vi "Z.vi"(8 "error in (no error)":errorcluster, 10 "Wire in":T1, 11 "Gate in":refnum<class "G-UE.lvclass">) -> (0 "error out":errorcluster, 3 "Gate out":refnum<class "G-UE.lvclass">)   [LabVIEW 2016, in "G-UE.lvclass"]
uses:
  G-UE.lvclass
  TypeDefs/Circuit Cluster.ctl
  GateAbst/GateAbst.lvclass
  <vilib>/Analysis/Matrix/Datatypes/ComplexMatrix.ctl
  <vilib>/Analysis/Matrix/NI_Matrix.lvlib
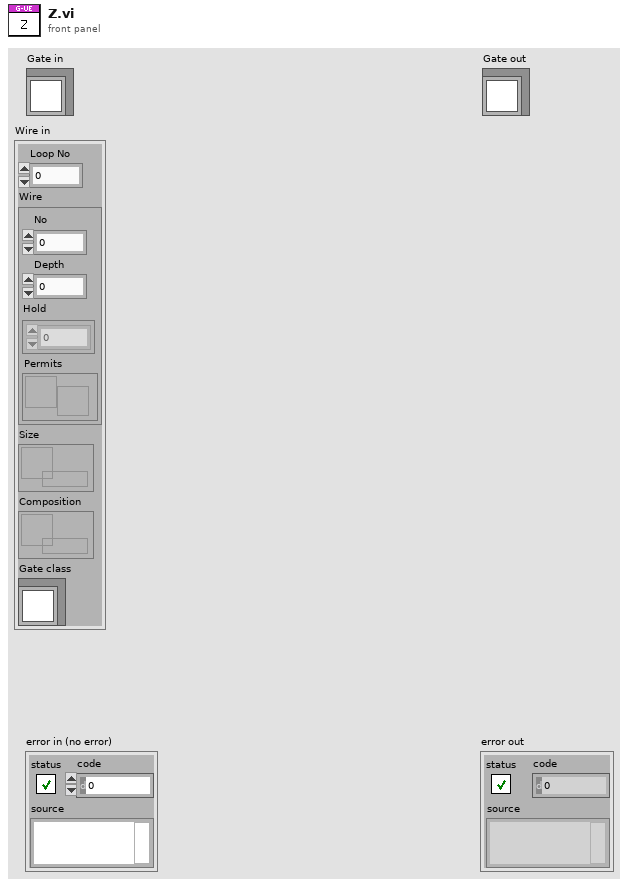
[diagram p1: front panel]
types:
  T1 = typedef "Circuit Cluster.ctl" = cluster{"Loop No":i32, "Wire":cluster{"No":i32, "Depth":i32, "Hold":i32[][], "Permits":refnum<notifier>}, "Size":refnum<queue>, "Composition":refnum<queue>, "Gate class":refnum<class "GateAbst.lvclass">}
  T2 = typedef "NI_Matrix.lvlib/ComplexMatrix.ctl" = cdb[][]
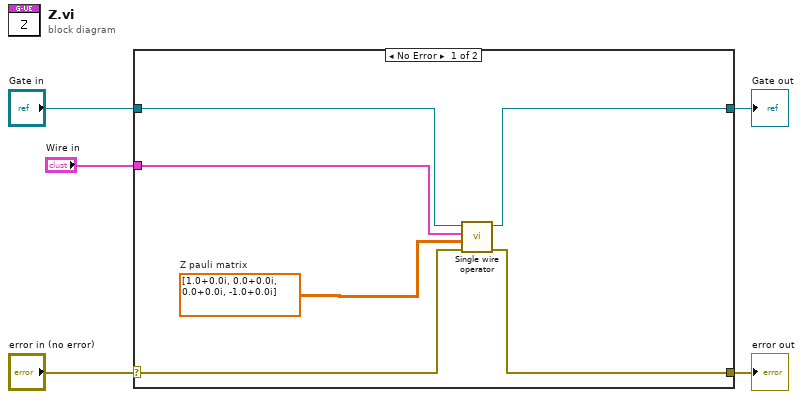
[diagram p0: block diagram]
diagram:
  n1 = case shown="No Error" "error in (no error)" {
    selector: "error in (no error)" -> [w7 w13]
    tunnel: [w9 w13] -> w4
    tunnel: [w10 w12] -> w2
    tunnel: "Gate in" -> [w11 w12]
    tunnel: "Wire in" -> [w6 _]
    frame No Error {
      w8 = T2 [[1.0+0.0i, 0.0+0.0i], [0.0+0.0i, -1.0+0.0i]]  # Z pauli matrix
      n2 = call "Single wire operator.vi"("error in (no error)"=w7, "Operator matrix"=w8, "Wire in"=w6, "G-UE in"=w11) -> ("error out"=w9:errorcluster, "G-UE out"=w10:refnum<class "G-UE.lvclass">)  [unwired: 6 in]
    }
    frame Error {
    }
  }
  "error out" <- w4
  "Gate out" <- w2
